vi "DialogBox.vi"(7 "Caption.Text":string) -> (2 "Output":bool)   [LabVIEW 2020]
panel:
  in  "Да":bool caption="Перезагрузить\nдетектор?"
  in  "Нет":bool
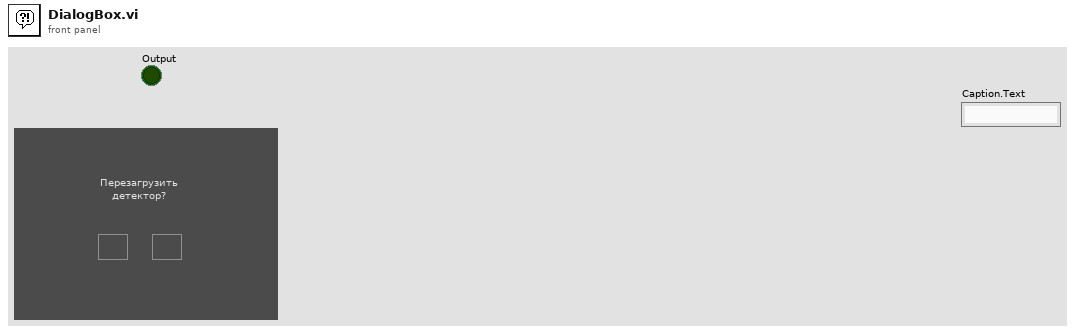
[diagram p1: front panel]
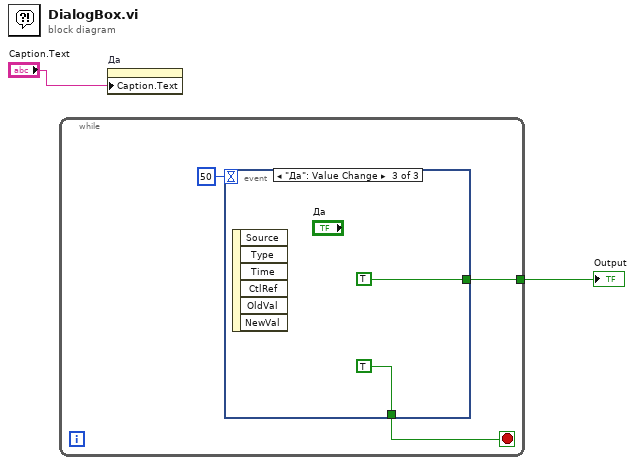
[diagram p0: block diagram]
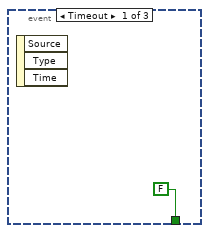
[diagram p2: hidden frame]
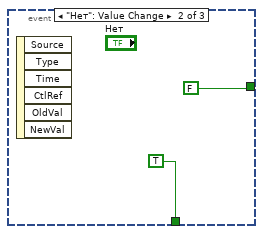
[diagram p3: hidden frame]
diagram:
  n1 = while {
    tunnel: [w4] -> w2
    stop <- w3 stop-if-true
    n2 = event shown="[2] \"Да\": Value Change" {
      selector: _ -> [_ _ _]
      dyn-events: _ -> [_ _ _]
      timeout: 50 -> [_ _ _]
      tunnel: [_ FALSE TRUE] -> w4
      tunnel: [FALSE TRUE TRUE] -> w3
      event Timeout {
        n3 = event-data() -> ()  [unwired: 1 in, 3 out]
      }
      event "Нет": Value Change {
        n4 = event-data() -> ()  [unwired: 1 in, 6 out]
      }
      event "Да": Value Change {
        n5 = event-data() -> ()  [unwired: 1 in, 6 out]
      }
    }
  }
  "Output" <- w2
  n6 = property on="Да" class="Bool"("Caption.Text"="Caption.Text") -> ()  [unwired: 2 in, 2 out]
